vi "MH_RotTTTRBuffer.vi"() -> ()   [LabVIEW 2019]
panel:
  out "Rotation Size":i32
  out "deltaT Rotate":u32
  out "NewWinIndex":i32
  in  "WinIndex":i32
  out "NewBuffIndex":i32
  in  "truetime":u64
  in  "Buffsize":i32
  in  "Buffindex":i32
  out "tableau (n rotations)":u64[](array[numeric])
  in  "Tableau":u64[](array[numeric])
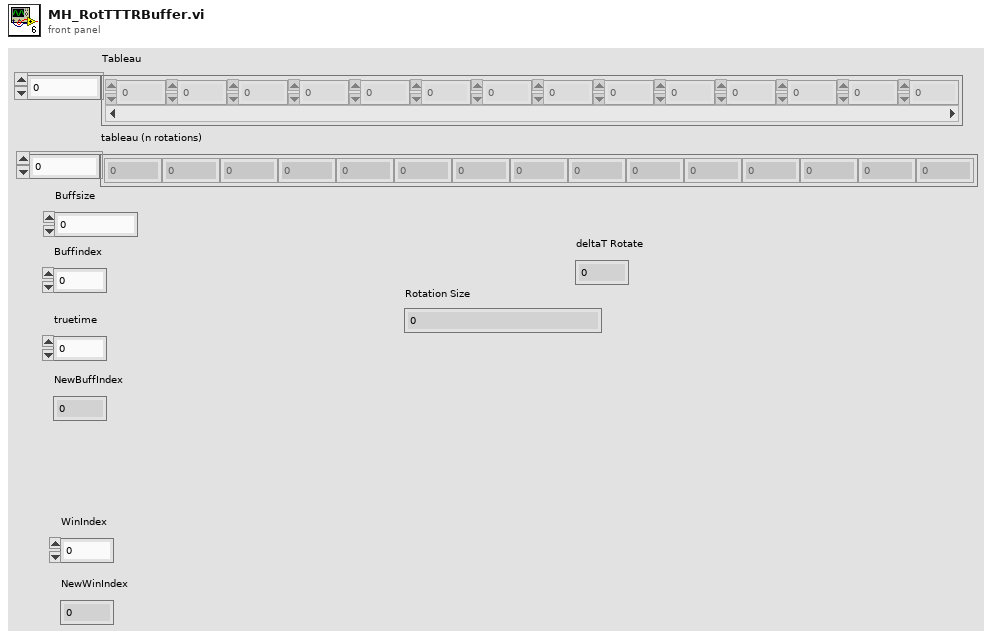
[diagram p1: front panel]
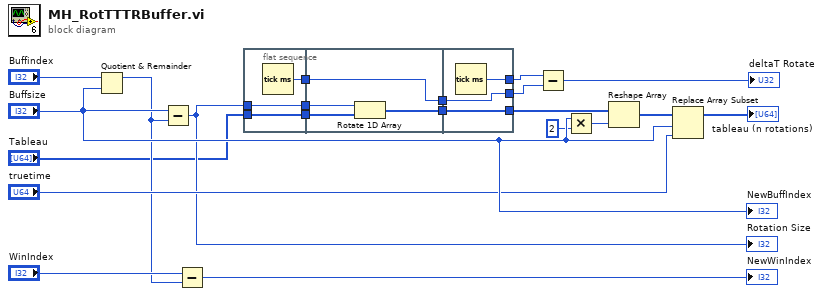
[diagram p0: block diagram]
diagram:
  n1 = Quotient & Remainder(x="Buffindex", y="Buffsize") -> (x-y*floor(x/y)=w14:i32)  [unwired: 1 out]
  n2 = Subtract(x="Buffsize", y=w14) -> (x-y=w16:i32)
  "Rotation Size" <- w16
  n3 = Subtract(x="WinIndex", y=w14) -> (x-y=→"NewWinIndex":i32)
  n4 = flat-sequence {
    tunnel: w16 -> [w23]
    tunnel: "Tableau" -> [w24]
    tunnel: [w24] -> w12
    tunnel: [w23] -> w11
    tunnel: [w22] -> w8
    tunnel: w12 -> [w27]
    tunnel: w11 -> [w26]
    tunnel: [w28] -> w10
    tunnel: [w25] -> w9
    tunnel: w8 -> [w25]
    tunnel: [w31] -> w21
    tunnel: w10 -> [w31]
    tunnel: [w30] -> w6
    tunnel: w9 -> [w30]
    tunnel: [w29] -> w7
    frame #0 {
      n5 = Tick Count (ms)() -> (millisecond timer value=w22:u32)
    }
    frame #1 {
      n6 = Rotate 1D Array(1:w27, 2:w26) -> (0:w28:u64[])
    }
    frame #2 {
      n7 = Tick Count (ms)() -> (millisecond timer value=w29:u32)
    }
  }
  n8 = Subtract(x=w7, y=w6) -> (x-y=→"deltaT Rotate":u32)
  n9 = Multiply(x="Buffsize", y=2) -> (x*y=w2:i32)
  n10 = Reshape Array(w21, w2) -> (w1:u64[])
  n11 = Replace Array Subset(array=w1, new element="truetime", index="Buffsize") -> (→"tableau (n rotations)":u64[])
  "NewBuffIndex" <- "Buffsize"
